vi "S2C_FORNAX_Proc_ManageVipFile.vi"(8 "Error In":errorcluster, 11 "Data In":string) -> (0 "Error Out":errorcluster, 3 "Data Out":string)   [LabVIEW 2015]
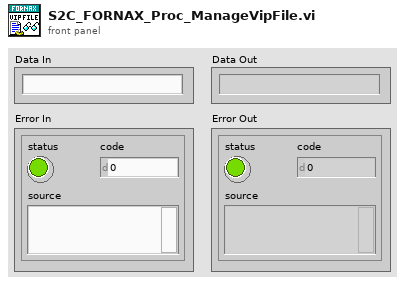
[diagram p1: front panel]
types:
  T1 = cluster{"Partition":string, "Message":string, "M_destId":i32, "M_message":string, "M_Crc32":i32}
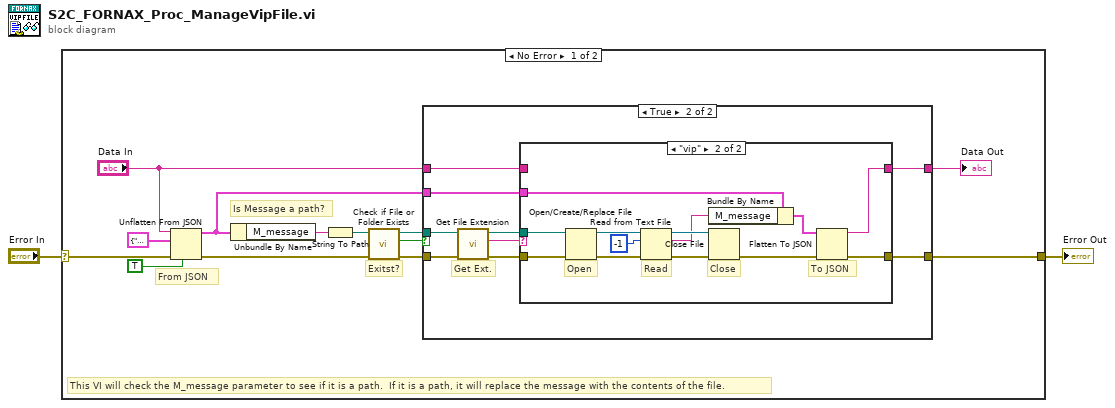
[diagram p0: block diagram]
diagram:
  n1 = case shown="No Error" "Error In" {
    selector: "Error In" -> [w13 w42]
    tunnel: [w5 w42] -> w1
    frame No Error {
      # "This VI will check the M_message parameter to see if it is a path.  If it is a path, it will replace the message with the contents of the file."
      # "Is Message a path?"
      # "Exitst?"
      # "From JSON"
      n2 = Unflatten From JSON(JSON string="Data In", type and defaults=T1 {"Partition"="", "Message"="", "M_destId"=0, "M_message"="", "M_Crc32"=0}, default null elements? (F)=TRUE, error in (no error)=w13) -> (value=w4:T1, error out=w12:errorcluster)  [unwired: 3 in]
      n3 = Unbundle By Name(w4) -> ("M_message"=w11:string)
      n4 = String To Path(string=w11) -> (path=w10:path)
      n5 = call <vilib>:"Check if File or Folder Exists.vi"("error in (no error)"=w12, "path"=w10) -> ("error out"=w9:errorcluster, "file or folder exists?"=w8:bool, "dup path"=w6:path)  [unwired: 7 in]
      n6 = case shown="True" w8 {
        tunnel: w9 -> [w16 w26]
        tunnel: "Data In" -> [w17 w18]
        tunnel: w6 -> [_ w25]
        tunnel: [w16 w21] -> w5
        tunnel: w4 -> [_ w20]
        tunnel: [w17 w19] -> w3
        frame False {
          # "Message is a command, not a path"
        }
        frame True {
          # "Get Ext."
          n7 = call <vilib>:"Get File Extension.vi"("error in (no error)"=w26, "file"=w25) -> ("error out"=w24:errorcluster, "lowercase file extension"=w23:string, "dup file"=w22:path)  [unwired: 5 in, 2 out]
          n8 = case shown="\"vip\"" w23 {
            tunnel: w24 -> [w27 w41]
            tunnel: w22 -> [_ w40]
            tunnel: [w27 w30] -> w21
            tunnel: w20 -> [_ w34]
            tunnel: [w28 w29] -> w19
            tunnel: w18 -> [w28 _]
            frame "Other", Default {
              # "File does not have a .vip extension"
            }
            frame "vip" {
              # "To JSON"
              # "Close"
              # "Read"
              # "Open"
              n9 = Open/Create/Replace File(file path (use dialog)=w40, error in=w41) -> (refnum out=w37:refnum<file>, error out=w39:errorcluster)  [unwired: 4 in, 1 out]
              n10 = Read from Text File(file (use dialog)=w37, count=-1, error in=w39) -> (refnum out=w35:refnum<file>, text=w33:string, error out=w36:errorcluster)  [unwired: 1 in, 1 out]
              n11 = Bundle By Name(cluster=w34, "M_message"=w33) -> (w31:T1)
              n12 = Close File(refnum=w35, error in=w36) -> (error out=w32:errorcluster)  [unwired: 1 out]
              n13 = Flatten To JSON(anything=w31, error in (no error)=w32) -> (JSON string=w29:string, 11:w30:errorcluster)  [unwired: 1 in]
            }
          }
        }
      }
      "Data Out" <- w3
    }
    frame Error {
    }
  }
  "Error Out" <- w1
